vi "initListenData.vi"(8 "error in (no error)":errorcluster) -> (0 "error out":errorcluster)   [LabVIEW 2017, in "communicateMLC.lvlib"]
uses:
  communicateMLC.lvlib
  TypeDefs/UDPListenFGV.ctl
  SubVIs/FGVs/TypeDefs/DataFGVControl.ctl
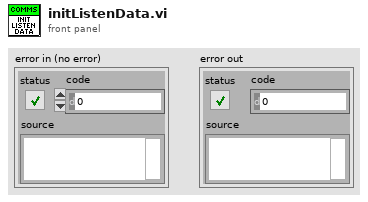
[diagram p1: front panel]
types:
  T1 = typedef "communicateMLC.lvlib/UDPListenFGV.ctl" = enum16{"Write", "Read"}
  T2 = typedef "DataFGVControl.ctl" = enum16{"init", "Set DataOut", "Get DataOut", "Set DataIn", "Get DataIn"}
  T3 = typedef "dataIn.ctl" = cluster{"Xtarget":dbl, "Ytarget":dbl, "Ztarget":dbl, "X_Attractor1":dbl, "Y_Attractor1":dbl, "Z_Attractor1":dbl, "X_Attractor2":dbl, "Y_Attractor2":dbl, "Z_Attractor2":dbl, "Traj_Flag":bool, "DeadZone":dbl, "Assistance":bool, "Shutdown":bool, "AssistanceLevel":dbl}
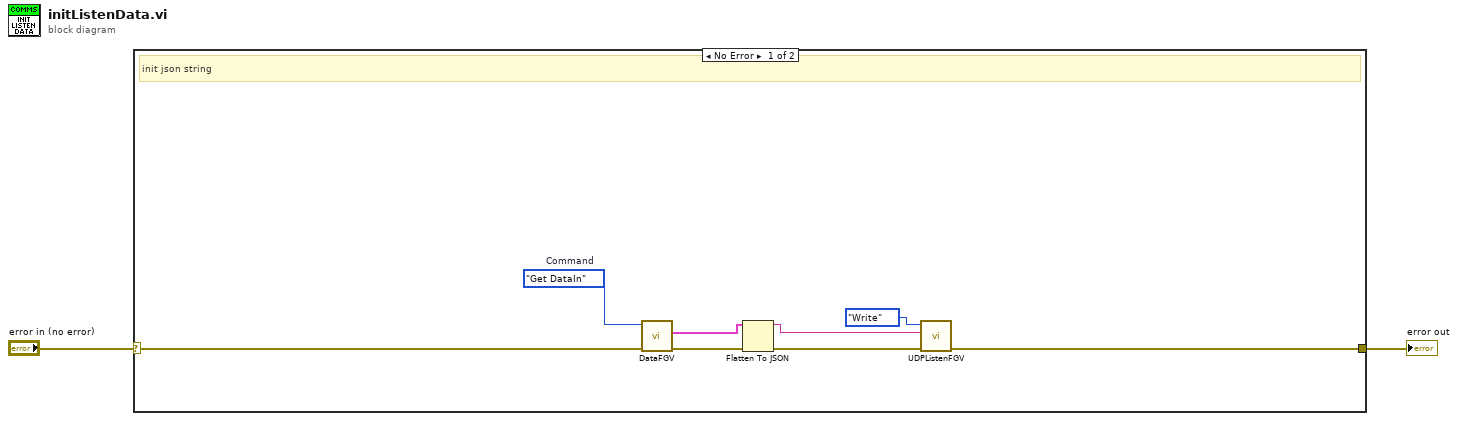
[diagram p0: block diagram]
diagram:
  n1 = case shown="No Error" "error in (no error)" {
    selector: "error in (no error)" -> [w8 w11]
    tunnel: [w10 w11] -> w2
    frame No Error {
      w7 = DataFGVControl."Get DataIn"  # Command
      # "init json string"
      n2 = call "DataFGV.vi"("error in (no error)"=w8, "Command"=w7) -> ("error out"=w6:errorcluster, "DataIn"=w4:T3)  [unwired: 7 in, 1 out]
      n3 = Flatten To JSON(anything=w4, error in (no error)=w6) -> (JSON string=w3:string, 11:w5:errorcluster)  [unwired: 1 in]
      n4 = call "UDPListenFGV.vi"("error in (no error)"=w5, "Write Data"=w3, "Command"=UDPListenFGV."Write") -> ("error out"=w10:errorcluster)  [unwired: 7 in, 1 out]
    }
    frame Error {
    }
  }
  "error out" <- w2
